vi "getStatusMovingAllAxes.vi"(0 "connection ID":i32, 5 "error in":errorcluster) -> (14 "connection ID":i32, 15 "moving1":i32, 16 "moving2":i32, 17 "moving3":i32, 19 "error out":errorcluster)   [LabVIEW 2016]
doc: "Get Status of all axes, see getStatusMoving for coding of the values"
panel:
  out "params_cluster":cluster{"Numeric":i32}
  in  "Params_cluster":cluster{"Numeric":dbl}
  in  "results_cluster":T1
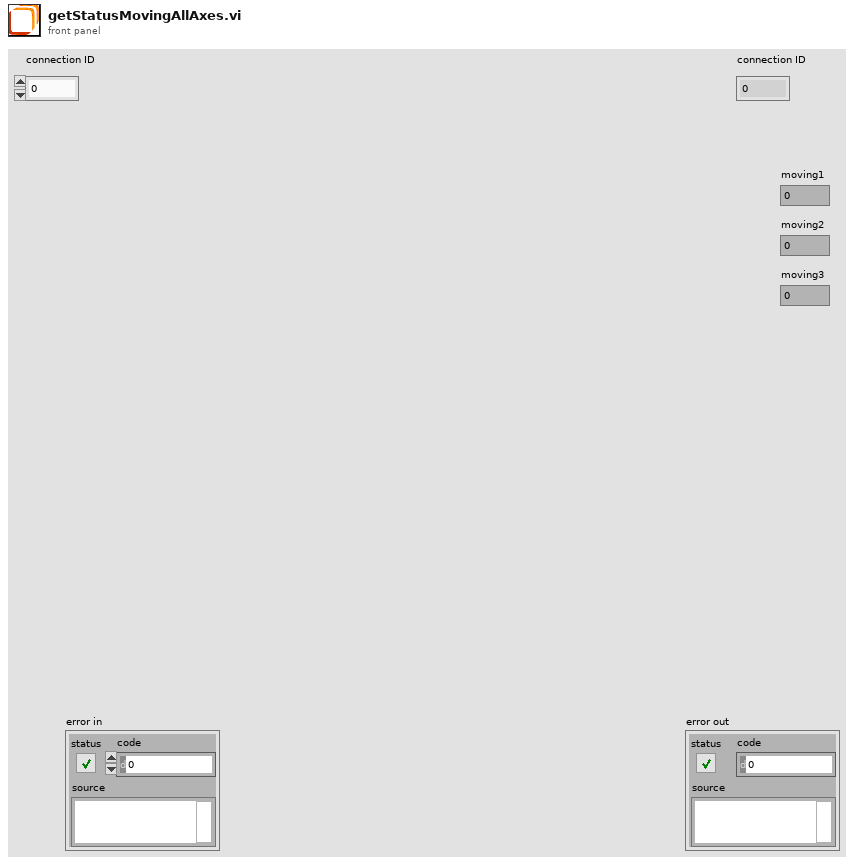
[diagram p1: front panel]
types:
  T1 = cluster{"errNo":i32, "moving1":i32, "moving2":i32, "moving3":i32}
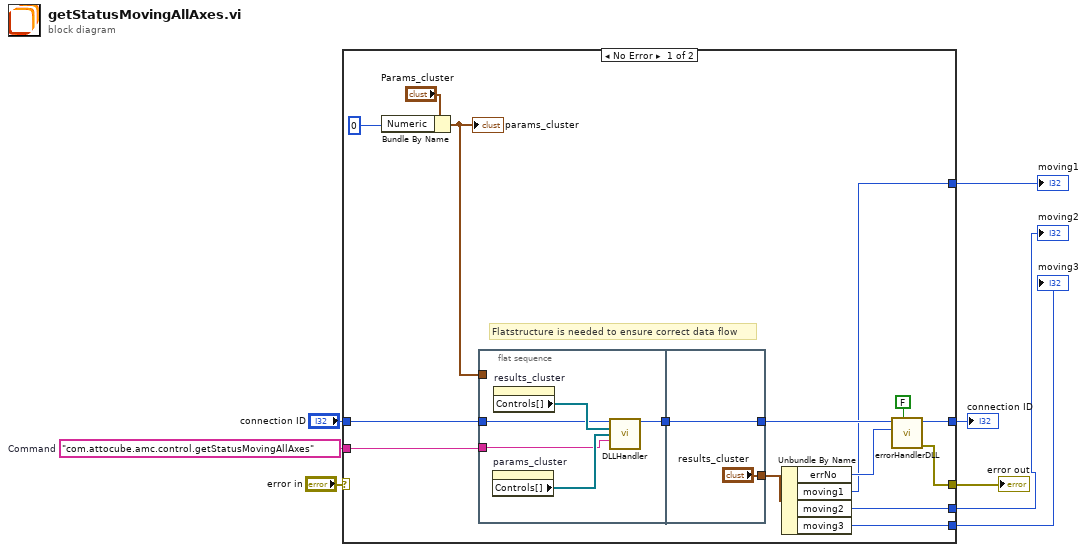
[diagram p0: block diagram]
diagram:
  w6 = "com.attocube.amc.control.getStatusMovingAllAxes"  # Command
  n1 = case shown="No Error" "error in" {
    selector: "error in" -> [_ w32]
    tunnel: [w22 w32] -> w8
    tunnel: w6 -> [w17 _]
    tunnel: [w16 w31] -> w5
    tunnel: "connection ID" -> [w15 w31]
    tunnel: [w11 _] -> w3
    tunnel: [w10 _] -> w2
    tunnel: [w9 _] -> w1
    frame No Error {
      # "Flatstructure is needed to ensure correct data flow"
      n2 = Bundle By Name(cluster="Params_cluster", "Numeric"=0) -> (w13:cluster{"Numeric":dbl})
      "params_cluster" <- w13
      n3 = flat-sequence {
        tunnel: [w28] -> w19
        tunnel: w17 -> [w25]
        tunnel: w15 -> [w24]
        tunnel: w13 -> [_]
        tunnel: ["results_cluster"] -> w20
        tunnel: [w30] -> w21
        tunnel: w19 -> [w30]
        frame #0 {
          n4 = property on="params_cluster" class="Clust (strict)"() -> ("Controls[]"=w26:refnum<vi>[])  [unwired: 2 in, 2 out]
          n5 = property on="results_cluster" class="Clust (strict)"() -> ("Controls[]"=w27:refnum<vi>[])  [unwired: 2 in, 2 out]
          n6 = call "DLLHandler.vi"("connection ID"=w24, "results_cluster"=w27, "params_cluster"=w26, "method"=w25) -> ("connection ID out"=w28:i32)  [unwired: 10 in, 1 out]
        }
        frame #1 {
        }
      }
      n7 = Unbundle By Name(w20) -> ("errNo"=w14:i32, "moving1"=w11:i32, "moving2"=w10:i32, "moving3"=w9:i32)
      n8 = call "errorHandlerDLL.vi"("show popup"=FALSE, "error number"=w14, "connection ID"=w21) -> ("error out"=w22:errorcluster, "connection ID"=w16:i32)  [unwired: 7 in]
    }
    frame Error {
    }
  }
  "error out" <- w8
  "connection ID" <- w5
  "moving1" <- w3
  "moving2" <- w2
  "moving3" <- w1
